vi "ramp_usage.vi"() -> ()   [LabVIEW 2018]
panel:
  out "Waveform Chart":i32(graph)
  out "Output":i32
  in  "Reset":bool
  in  "Continue":bool
  in  "Ramp 2 Time":dbl=5.0
  in  "Ramp 1 Time":dbl=20.0
  in  "Steady State":dbl=80.0
  in  "Standby":dbl=40.0
  in  "Start":dbl
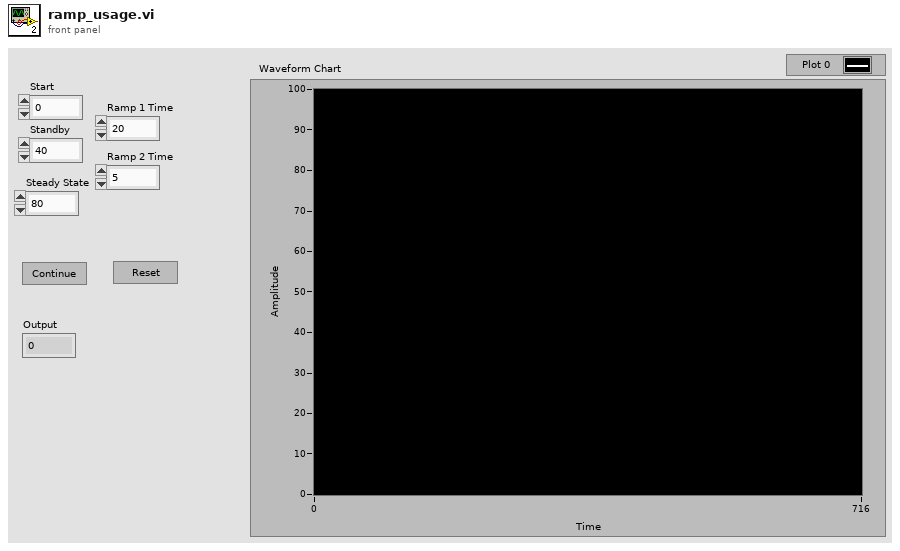
[diagram p1: front panel]
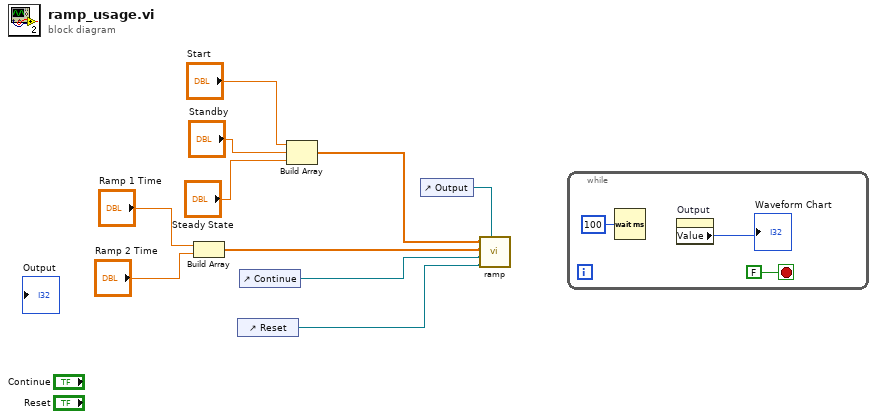
[diagram p0: block diagram]
diagram:
  n1 = Build Array("Ramp 1 Time", "Ramp 2 Time") -> (w4:dbl[])
  n2 = control-ref of="Reset"() -> (w2:refnum<vi>)
  n3 = control-ref of="Continue"() -> (w3:refnum<vi>)
  n4 = Build Array("Start", "Standby", "Steady State") -> (w5:dbl[])
  n5 = control-ref of="Output"() -> (w1:refnum<vi>)
  n6 = call "ramp.vi"("DigNum Refnum"=w1, "Bool Refnum Reset"=w2, "Bool Refnum Start"=w3, "Time Per Step"=w4, "Pressures"=w5) -> ()  [unwired: 4 in]
  n7 = while {
    stop <- FALSE stop-if-true
    n8 = Wait (ms)(milliseconds to wait=u32 100) -> ()  [unwired: 1 out]
    n9 = property on="Output" class="DigNum (strict)"() -> ("Value"=→"Waveform Chart":i32)  [unwired: 2 in, 2 out]
  }
